vi "Remove Variable.vi"(8 "error in (no error)":errorcluster, 9 "Name":string, 10 "Variable Type":enum16{"Project", "Execution"}(ring), 11 "Project in":refnum<class "Project.lvclass">) -> (0 "error out":errorcluster, 3 "Project out":refnum<class "Project.lvclass">)   [LabVIEW 2015, in "Project.lvclass"]
uses:
  Project.lvclass
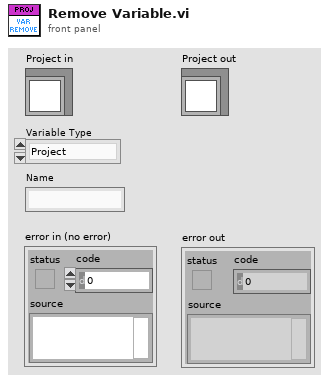
[diagram p1: front panel]
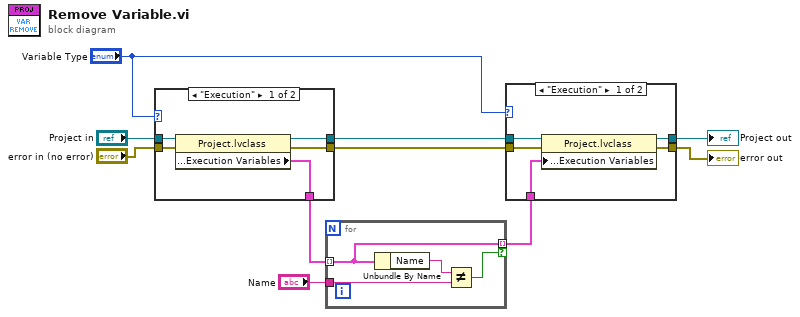
[diagram p0: block diagram]
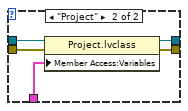
[diagram p2: hidden frame]
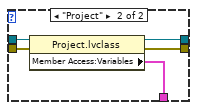
[diagram p3: hidden frame]
diagram:
  n1 = case shown="\"Execution\"" "Variable Type" {
    tunnel: "Project in" -> [w15 w20]
    tunnel: [w14 w19] -> w9
    tunnel: [w13 w18] -> w7
    tunnel: "error in (no error)" -> [w12 w17]
    tunnel: [w11 w16] -> w4
    frame "Execution" {
      n2 = property class="Project.lvclass"(reference=w15, error in=w12) -> (reference out=w13:refnum<class "Project.lvclass">, error out=w11:errorcluster, "Member Access:Execution Variables"=w14:cluster{"Name":string, "Value":variant}[])
    }
    frame "Project" {
      n3 = property class="Project.lvclass"(reference=w20, error in=w17) -> (reference out=w18:refnum<class "Project.lvclass">, error out=w16:errorcluster, "Member Access:Variables"=w19:cluster{"Name":string, "Value":variant}[])
    }
  }
  n4 = for {
    tunnel: w9 -> [w22] mode=indexing
    tunnel: "Name" -> [w23]
    tunnel: [w22] -> w6 mode=indexing if=w21
    n5 = Unbundle By Name(w22) -> ("Name"=w24:string)
    n6 = Not Equal?(x=w24, y=w23) -> (x != y?=w21:bool)
  }
  n7 = case shown="\"Execution\"" "Variable Type" {
    tunnel: w7 -> [w29 w34]
    tunnel: w6 -> [w28 w33]
    tunnel: w4 -> [w27 w32]
    tunnel: [w26 w31] -> w3
    tunnel: [w25 w30] -> w2
    frame "Execution" {
      n8 = property class="Project.lvclass"(reference=w29, error in=w27, "Member Access:Execution Variables"=w28) -> (reference out=w26:refnum<class "Project.lvclass">, error out=w25:errorcluster)
    }
    frame "Project" {
      n9 = property class="Project.lvclass"(reference=w34, error in=w32, "Member Access:Variables"=w33) -> (reference out=w31:refnum<class "Project.lvclass">, error out=w30:errorcluster)
    }
  }
  "error out" <- w2
  "Project out" <- w3
